vi "Compute Turns(3pt).vi"(9 "Long Offset":dbl, 10 "Mid Offset":dbl, 11 "Short Offset":dbl) -> (3 "Turns Clockwise":dbl format="%.3f")   [LabVIEW 2019]
uses:
  <vilib>/Analysis/6fits.llb/Curve Fitting Criteria.ctl
  Analysis/Global Tube Measurement.vi
  <vilib>/Analysis/NI_AALPro.lvlib
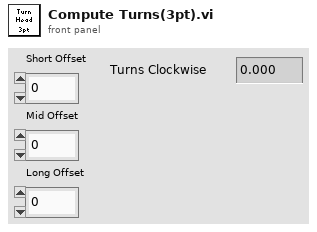
[diagram p1: front panel]
types:
  T1 = typedef "NI_AALPro.lvlib/Curve Fitting Criteria.ctl" = u16
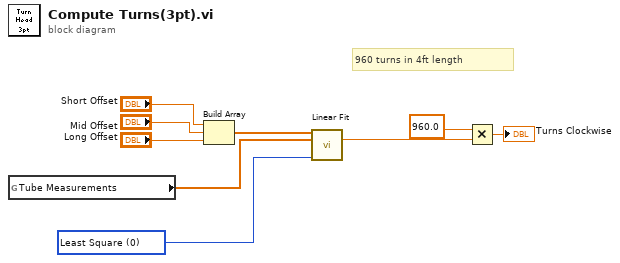
[diagram p0: block diagram]
diagram:
  w2 = T1 0 items=["Least Square", "Least Absolute Residual", "Bisquare"] ("method")
  # "960 turns in 4ft length"
  n1 = global read "Global Tube Measurement.vi" "Tube Measurements"() -> (w1:dbl[])
  n2 = Build Array("Short Offset", "Mid Offset", "Long Offset") -> (w6:dbl[])
  n3 = call <vilib>:"Linear Fit.vi"("Y"=w6, "X"=w1, "method"=w2) -> ("slope"=w8:dbl)  [unwired: 8 in, 4 out]
  n4 = Multiply(x=960.0 ("Offset 3"), y=w8) -> (x*y=→"Turns Clockwise":dbl)
